vi "first file.vi"() -> ()   [LabVIEW 2012]
panel:
  out "Array":dbl[][](array[numeric])
  in  "stop":bool
  in  "access (0:read/write)":enum16{"read/write", "read-only", "write-only"}(ring)
  out "error out":errorcluster
  in  "operation (0:open)":T1(ring)
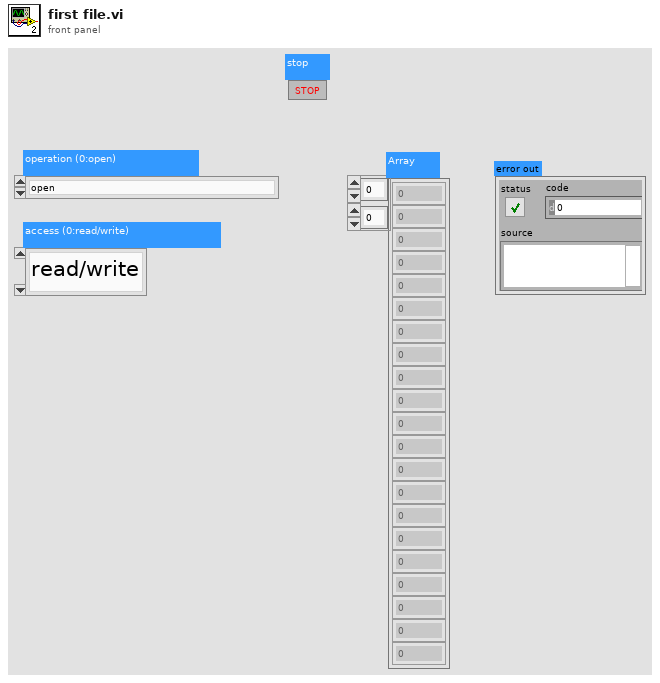
[diagram p1: front panel]
types:
  T1 = enum16{"open", "replace", "create", "open or create", "replace or create", "replace or create with confirmation"}
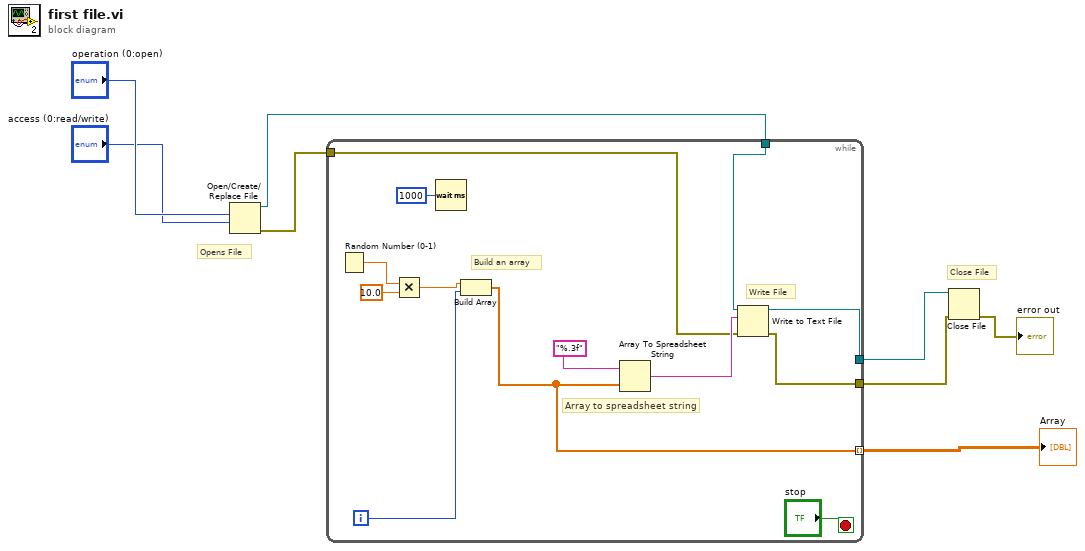
[diagram p0: block diagram]
diagram:
  # "Close File"
  # "Opens File"
  n1 = Open/Create/Replace File(operation (0:open)="operation (0:open)", access (0:read/write)="access (0:read/write)") -> (refnum out=w5:refnum<file>, error out=w3:errorcluster)  [unwired: 4 in, 1 out]
  n2 = while {
    tunnel: w5 -> [w16]
    tunnel: [w14] -> w4
    tunnel: w3 -> [w13]
    tunnel: [w12] -> w2
    tunnel: [w9] -> w1 mode=indexing
    i -> [w10]
    stop <- "stop" stop-if-true
    # "Write File"
    # "Array to spreadsheet string"
    # "Build an array"
    n3 = Random Number (0-1)() -> (number: 0 to 1=w20:dbl)
    n4 = Multiply(x=w20, y=10.0) -> (x*y=w11:dbl)
    n5 = Wait (ms)(milliseconds to wait=u32 1000) -> ()  [unwired: 1 out]
    n6 = Build Array(w11, w10) -> (w9:dbl[])
    n7 = Array To Spreadsheet String(array=w9, 3:"%.3f" ("format string")) -> (spreadsheet string=w17:string)  [unwired: 1 in]
    n8 = Write to Text File(file (use dialog)=w16, text=w17, error in=w13) -> (refnum out=w14:refnum<file>, error out=w12:errorcluster)  [unwired: 1 in, 1 out]
  }
  "Array" <- w1
  n9 = Close File(refnum=w4, error in=w2) -> (error out=→"error out":errorcluster)  [unwired: 1 out]
